vi "Open Subscription Policy.vi"(10 "Transport":refnum<class "ITransport.lvclass">, 11 "SubscriptionPolicy":refnum<class "BasicSubscription.lvclass">) -> (0 "error out":errorcluster, 3 "Subscription Policy":T1)   [LabVIEW 2015]
doc: "<License>\nCopyright © 2017 Composed Systems, LLC | All rights reserved\nwww.composed.io\n\nAuthor: Ethan Stern <ethan.stern@composed.io>\n\nThis software is provided \"AS IS\" WITHOUT WARRANTIES, either express or implied, AND IS FOR EDUCATIONAL PURPOSES ONLY.\n</License>"
uses:
  BasicSubscription.lvclass
  IMediator/ITransport/ITransport.lvclass
  ISubscriptionPolicy Reference.ctl
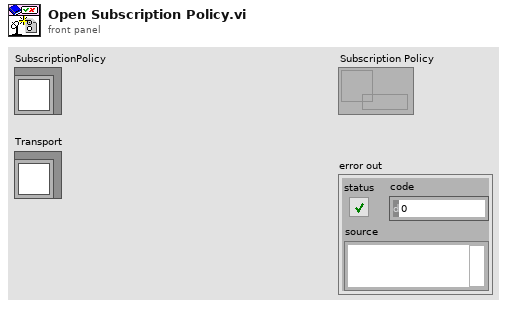
[diagram p1: front panel]
types:
  T1 = typedef "ISubscriptionPolicy Reference.ctl" = refnum<data-value>
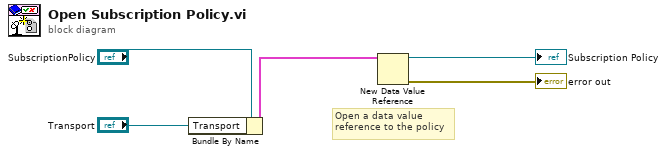
[diagram p0: block diagram]
diagram:
  # "Open a data value\nreference to the policy"
  n1 = Bundle By Name(cluster="SubscriptionPolicy", "Transport"="Transport") -> (w2:cluster{})
  n2 = New Data Value Reference(data value=w2) -> (data value reference=→"Subscription Policy":refnum<data-value>, error out=→"error out":errorcluster)  [unwired: 1 in]
